vi "FTW-JSON-Construct-FromBuffer.vi"(5 "JSON String (UTF-8)":string, 11 "error in":errorcluster) -> (4 "JSON Object":refnum<data-value>, 15 "error out":errorcluster)   [LabVIEW 2014]
uses:
  core/FTW-JSON-Core-Structure.ctl
  error/FTW-ERR-NoErrorConstant.vi
  error/FTW-ERR-CallChain.vi
  string/FTW-STR-ReplaceWhitespace.vi
panel:
  # "Inputs"
  # "Outputs"
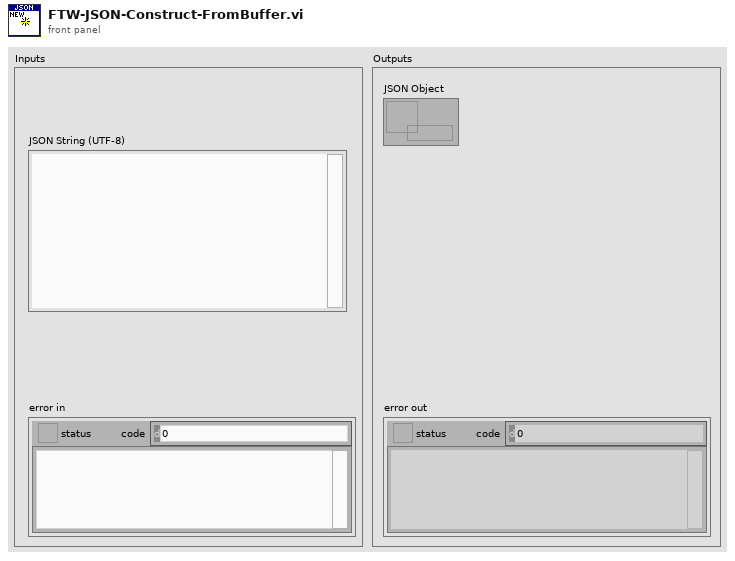
[diagram p1: front panel]
types:
  T1 = typedef "FTW-JSON-Core-Structure.ctl" = cluster{"JSON Object":i64, "Encoding Flags":i64, "Decoding Flags":i64}
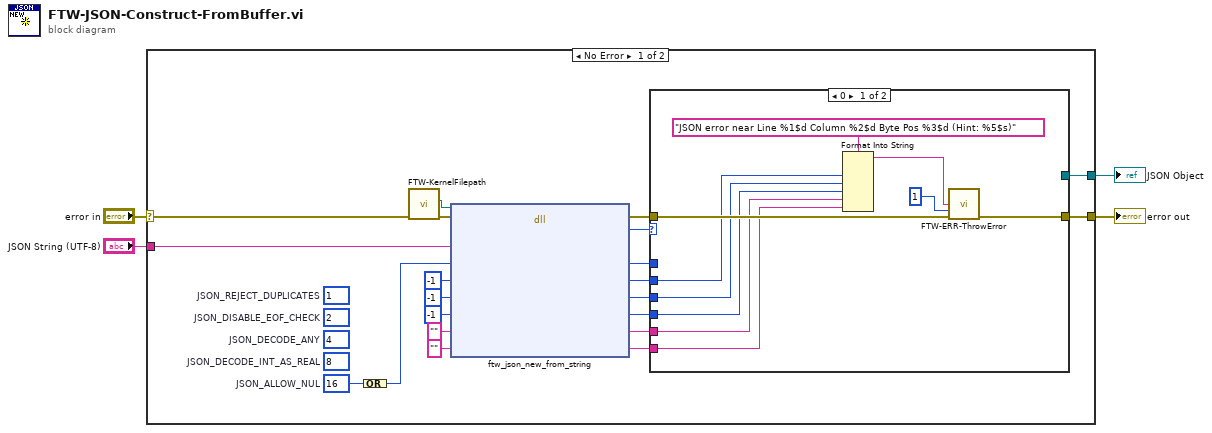
[diagram p0: block diagram]
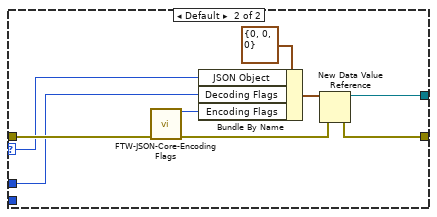
[diagram p2: hidden frame]
diagram:
  n1 = case shown="No Error" "error in" {
    selector: "error in" -> [w7 w45]
    tunnel: [w23 w45] -> w4
    tunnel: [w24 _] -> w1
    tunnel: "JSON String (UTF-8)" -> [w22 _]
    frame No Error {
      w25 = i64 16  # JSON_ALLOW_NUL
      (unwired) i64 8  # JSON_DECODE_INT_AS_REAL
      (unwired) i64 4  # JSON_DECODE_ANY
      (unwired) i64 2  # JSON_DISABLE_EOF_CHECK
      (unwired) i64 1  # JSON_REJECT_DUPLICATES
      n2 = Compound Arithmetic op=OR(w25) -> (w20:i64)
      n3 = call "FTW-KernelFilepath.vi"("error in"=w7) -> ("error out"=w6:errorcluster, "Library Filepath"=w5:path)  [unwired: 8 in, 1 out]
      n4 = dll-call lib="?" fn="ftw_json_new_from_string"(path in=w5, error in=w6, "JSON Buffer"=w22, "Flags"=w20, "Error Line Number"=i64 -1, "Error Column Number"=i64 -1, "Error Byte Position"=i64 -1, "Error Source"="", "Error Hint"="") -> (error out=w21:errorcluster, "JSON Object Pointer"=w19:i64, "Flags"=w18:i64, "Error Line Number"=w17:i64, "Error Column Number"=w16:i64, "Error Byte Position"=w15:i64, "Error Source"=w14:string, "Error Hint"=w13:string)  [unwired: 2 in, 1 out]
      n5 = case shown="0" w19 {
        selector: w19 -> [_ w37]
        tunnel: [_ w42] -> w24
        tunnel: [w31 w41] -> w23
        tunnel: w21 -> [w32 w38]
        tunnel: w18 -> [_ w36]
        tunnel: w17 -> [w30 _]
        tunnel: w16 -> [w29 _]
        tunnel: w15 -> [w28 _]
        tunnel: w14 -> [w27 _]
        tunnel: w13 -> [w26 _]
        frame 0 {
          n6 = Format Into String(format string="JSON error near Line %1$d Column %2$d Byte Pos %3$d (Hint: %5$s)", w30, w29, w28, w27, w26) -> (resulting string=w34:string)  [unwired: 2 in, 1 out]
          n7 = call "FTW-ERR-ThrowError.vi"("Error Message"=w34, "Error Code"=1, "error in"=w32) -> ("error out"=w31:errorcluster)  [unwired: 12 in]
        }
        frame Default {
          n8 = call "FTW-JSON-Core-EncodingFlags.vi"("error in"=w38) -> ("Encoding Flags"=w40:i64, "error out"=w39:errorcluster)  [unwired: 13 in]
          n9 = Bundle By Name(cluster=T1 {"JSON Object"=0, "Encoding Flags"=0, "Decoding Flags"=0}, "JSON Object"=w37, "Decoding Flags"=w36, "Encoding Flags"=w40) -> (w43:T1)
          n10 = New Data Value Reference(data value=w43, error in=w39) -> (data value reference=w42:refnum<data-value>, error out=w41:errorcluster)
        }
      }
    }
    frame Error {
    }
  }
  "error out" <- w4
  "JSON Object" <- w1
